vi "Queue Actor.vi"(8 "Queue Caller":map{string, refnum<data-value>}(c390), 9 "Queue of Queue Self":refnum<queue>, 10 "Queue Self Alias":string, 11 "Queue Actor":refnum<class "Queue Actor.lvclass">) -> ()   [LabVIEW 2021, in "jettl.lvlib" / "Base Queue Actor.lvclass"]
uses:
  Base Queue Actor.lvclass
  Queue Actor/Queue Actor.lvclass
  C:/git/jettl/src/jettl/Actor/Actor.lvclass
  Msg/Msg/Msg.lvclass
  C:/git/jettl/src/jettl/Queue Actor/Queue Actor.lvclass
  Msg/Msgs/Queue Last Ack/Queue Last Ack Msg/Queue Last Ack Msg.lvclass
  C:/git/jettl/src/jettl/Msg/Msg.lvclass
  jettl.lvlib
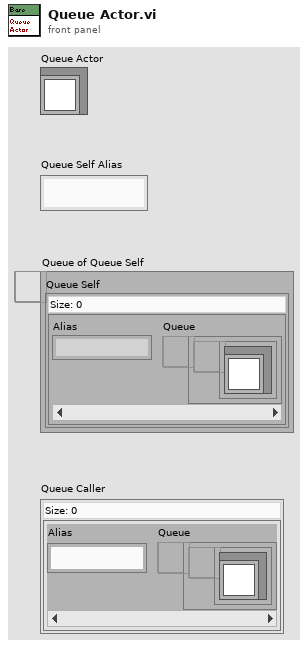
[diagram p1: front panel]
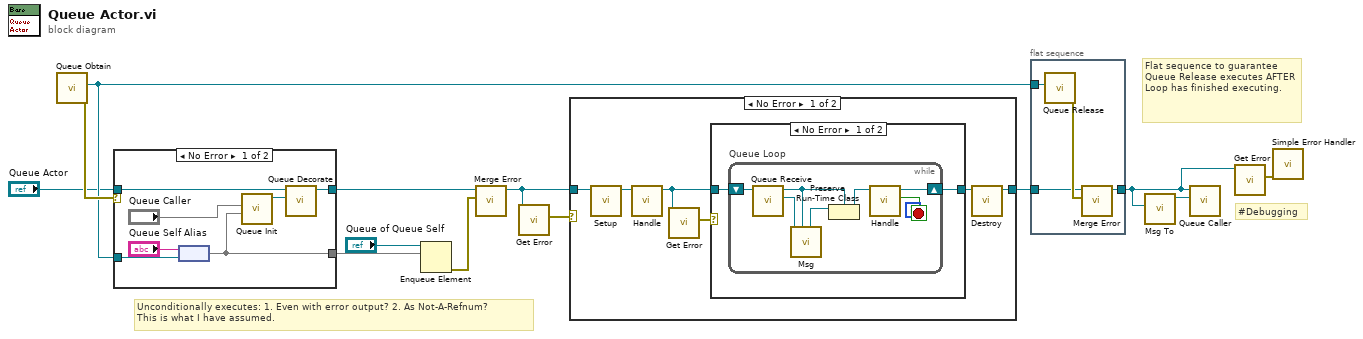
[diagram p0: block diagram]
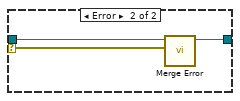
[diagram p2: hidden frame]
diagram:
  # "#Debugging"
  # "Flat sequence to guarantee Queue Release executes AFTER Loop has finished executing."
  # "Unconditionally executes: 1. Even with error output? 2. As Not-A-Refnum?\nThis is what I have assumed."
  n1 = call "Queue Obtain.vi"() -> ("error out"=w13:errorcluster, "Queue"=w9:refnum<data-value>)  [unwired: 10 in]
  n2 = case shown="No Error" w13 {
    selector: w13 -> [_ w22]
    tunnel: [w14 w23] -> w7
    tunnel: "Queue Actor" -> [w20 w21]
    tunnel: w9 -> [w17 _]
    tunnel: [w15 _] -> w6
    frame No Error {
      n3 = node("Queue Self Alias", w17) -> (w15:map{string, refnum<data-value>})
      n4 = call "Queue Init.vi"("Queue Self"=w15, "Queue Caller"="Queue Caller") -> ("Base Queue Actor out"=w19:refnum<class "Base Queue Actor.lvclass">)  [unwired: 9 in]
      n5 = call-dynamic "Queue Decorate.vi"("Queue Actor"=w19, "Queue Actor in"=w20) -> ("Queue Actor out"=w14:refnum<class "Queue Actor.lvclass">)  [unwired: 9 in]
    }
    frame Error {
      n6 = call-dynamic "Merge Error.vi"("Error"=w22, "Set Error in"=w21) -> ("Set Error out"=w23:refnum<class "Queue Actor.lvclass">)  [unwired: 9 in]
    }
  }
  n7 = Enqueue Element(queue="Queue of Queue Self", element=w6) -> (error out=w11:errorcluster)  [unwired: 2 in, 2 out]
  n8 = call-dynamic "Merge Error.vi"("Error"=w11, "Set Error in"=w7) -> ("Set Error out"=w12:refnum<class "Queue Actor.lvclass">)  [unwired: 9 in]
  n9 = call-dynamic "Get Error.vi"("Actor in"=w12) -> ("Error"=w5:errorcluster)  [unwired: 10 in]
  n10 = case shown="No Error" w5 {
    tunnel: w12 -> [w27 w40]
    tunnel: [w28 w40] -> w4
    frame No Error {
      n11 = call-dynamic "Setup.vi"("Setup in"=w27) -> ("Setup out"=w26:refnum<class "Queue Actor.lvclass">)  [unwired: 10 in]
      n12 = call-dynamic "Handle.vi"("Actor in"=w26) -> ("Actor out"=w24:refnum<class "Queue Actor.lvclass">)  [unwired: 9 in, 1 out]
      n13 = call-dynamic "Get Error.vi"("Actor in"=w24) -> ("Error"=w25:errorcluster)  [unwired: 10 in]
      n14 = case shown="No Error" w25 {
        tunnel: [w31 w39] -> w29
        tunnel: w24 -> [w30 w39]
        frame No Error {
          n15 = while "Queue Loop" {
            shift-right: [w38] -> w31
            shift-left: w30 -> [w37]
            stop <- w35 stop-if-true
            n16 = call-dynamic "Queue Receive.vi"("Queue Actor in"=w37) -> ("Msg"=w36:refnum<class "Msg.lvclass">, "Queue Actor out"=w34:refnum<class "Queue Actor.lvclass">)  [unwired: 9 in]
            n17 = call-dynamic "Msg.vi"("Actor in"=w34, "Msg in"=w36) -> ("Actor out"=w32:refnum<class "Actor.lvclass">)  [unwired: 9 in]
            n18 = Preserve Run-Time Class(object in=w32, 2:w34) -> (object out=w33:refnum<class "Queue Actor.lvclass">)  [unwired: 1 in, 1 out]
            n19 = call-dynamic "Handle.vi"("Actor in"=w33) -> ("Destroy?"=w35:bool, "Actor out"=w38:refnum<class "Queue Actor.lvclass">)  [unwired: 9 in]
          }
        }
        frame Error {
        }
      }
      n20 = call-dynamic "Destroy.vi"("Actor in"=w29) -> ("Actor out"=w28:refnum<class "Queue Actor.lvclass">)  [unwired: 10 in]
    }
    frame Error {
    }
  }
  n21 = flat-sequence {
    tunnel: w9 -> [w44]
    tunnel: [w43] -> w1
    tunnel: w4 -> [w41]
    frame #0 {
      n22 = call "Queue Release.vi"("Queue"=w44) -> ("error out"=w42:errorcluster)  [unwired: 10 in]
      n23 = call-dynamic "Merge Error.vi"("Error"=w42, "Set Error in"=w41) -> ("Set Error out"=w43:refnum<class "Queue Actor.lvclass">)  [unwired: 9 in]
    }
  }
  n24 = call "Msg To.vi"("Queue Actor"=w1) -> ("Queue Last Ack Msg out"=w3:refnum<class "Queue Last Ack Msg.lvclass">)  [unwired: 10 in]
  n25 = call-dynamic "Queue Caller.vi"("Msg"=w3, "Actor in"=w1) -> ()  [unwired: 9 in, 1 out]
  n26 = call-dynamic "Get Error.vi"("Actor in"=w1) -> ("Error"=w2:errorcluster)  [unwired: 10 in]
  n27 = call <vilib>:"Simple Error Handler.vi"("error in (no error)"=w2) -> ()  [unwired: 4 in, 5 out]
